vi "Terminal Type Matches Pattern.vi"(5 "Enum Names ?":bool, 7 "Include Names":bool, 8 "error in (no error)":errorcluster, 10 "Terminal Type Pattern":string, 11 "Terminal":T1) -> (0 "error out":errorcluster, 3 "Terminal Matches Pattern ?":bool)   [LabVIEW 2018, in "Scripting Tools.lvlib" / "XNode Support.lvlib"]
doc: "Tests whether ther data type for <b>Terminal</b> has a string representation that matches a regular expression pattern <b>Terminal Type Pattern</b>. The options <b>Include Names</b> and <b>Enum names ?</b> are used to determine whether the type representations tring includes element names and enum labels."
uses:
  XNode Support.lvlib
  <vilib>/XNodeSupport/XNodeTermIDPair.ctl
  <vilib>/XNodeSupport/XNodeTermRef.ctl
  <vilib>/XNodeSupport/XNodeString.ctl
  <vilib>/XNodeSupport/NI_XNodeSupport.lvlib
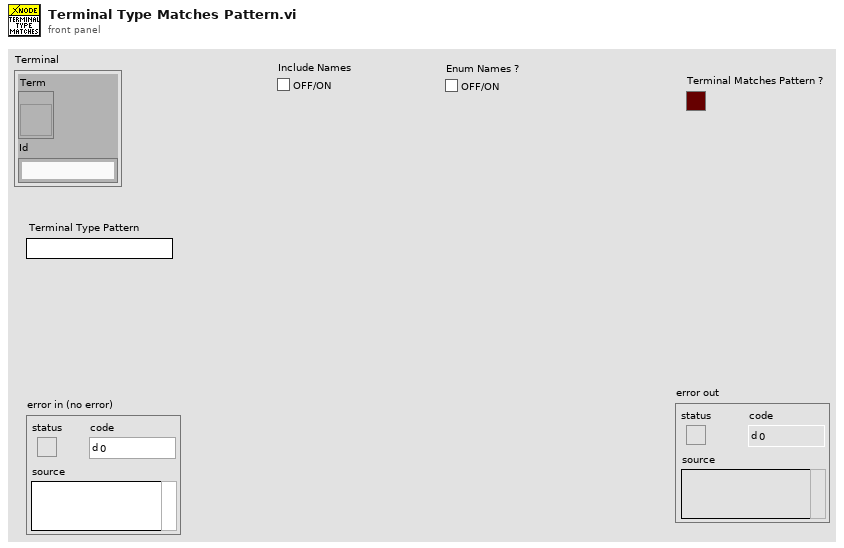
[diagram p1: front panel]
types:
  T1 = typedef "NI_XNodeSupport.lvlib/XNodeTermIDPair.ctl" = cluster{"Term":T2, "Id":T3}
  T2 = typedef "NI_XNodeSupport.lvlib/XNodeTermRef.ctl" = refnum<vi>
  T3 = typedef "NI_XNodeSupport.lvlib/XNodeString.ctl" = string
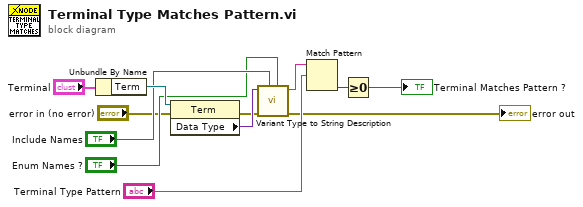
[diagram p0: block diagram]
diagram:
  n1 = Unbundle By Name("Terminal") -> ("Term"=w11:T2)
  n2 = property class="Term"(reference=w11, error in="error in (no error)") -> (error out=w9:errorcluster, "Data Type"=w10:variant)  [unwired: 1 out]
  n3 = call "Variant Type to String Description.vi"("Enum Names ?"="Enum Names ?", "Include Names"="Include Names", "error in (no error)"=w9, "Data Type"=w10) -> ("error out"=→"error out":errorcluster, "String Representation of Type"=w5:string)  [unwired: 5 in, 1 out]
  n4 = Match Pattern(string=w5, regular expression="Terminal Type Pattern") -> (offset past match=w2:i32)  [unwired: 1 in, 3 out]
  n5 = Greater Or Equal To 0?(x=w2) -> (x >= 0?=→"Terminal Matches Pattern ?":bool)
